vi "Bank of Parallel Filters.vi"() -> ()   [LabVIEW 2025]
uses:
  <vilib>/Analysis/1siggen.llb/Ramp Pattern by Samples.vi
  <vilib>/Analysis/2dsp.llb/Complex FFT.vi
  <vilib>/Analysis/baseanly.llb/Mean (CDB).vi
  <vilib>/Analysis/NI_AALPro.lvlib
  <vilib>/Analysis/NI_AALBase.lvlib
panel:
  in  "Cylcles Per Period":dbl=13.0 min=0.0 max=200.0 format="%#_13g"
  in  "Active Percent":dbl=100.0 min=0.0 max=100.0 step=1.0 format="%03.0f"
  in  "Offset":i32 min=0 max=100 step=1
  out "The Signal":dbl[](graph)
  out "The Spectrum":dbl[](graph)
  out "Parralell Filters":dbl[](graph)
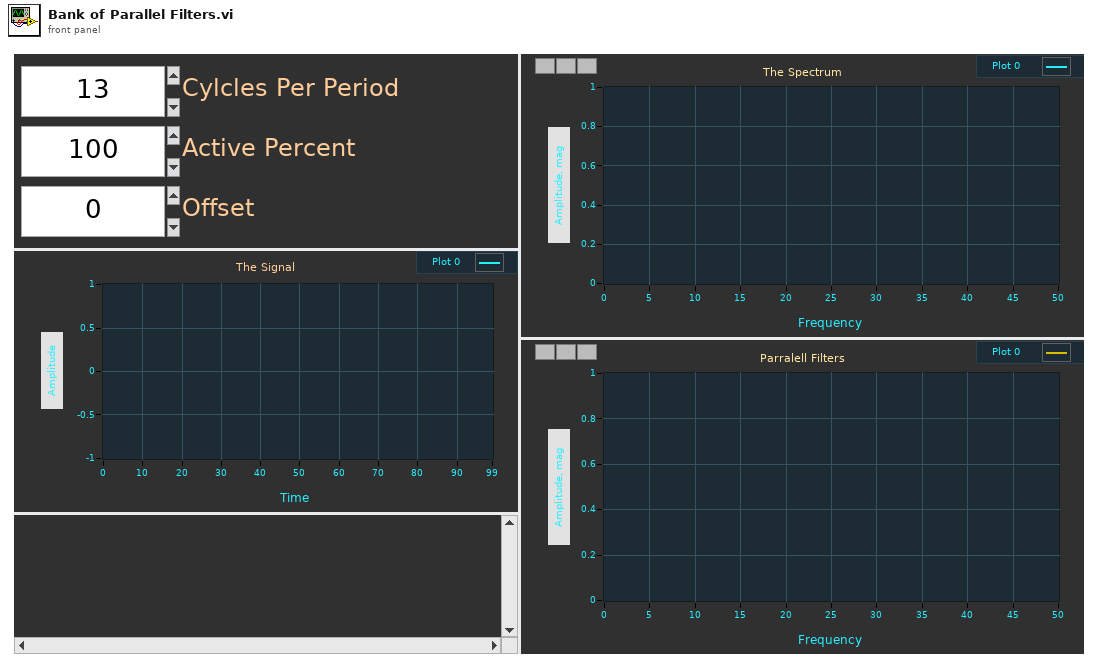
[diagram p1: front panel]
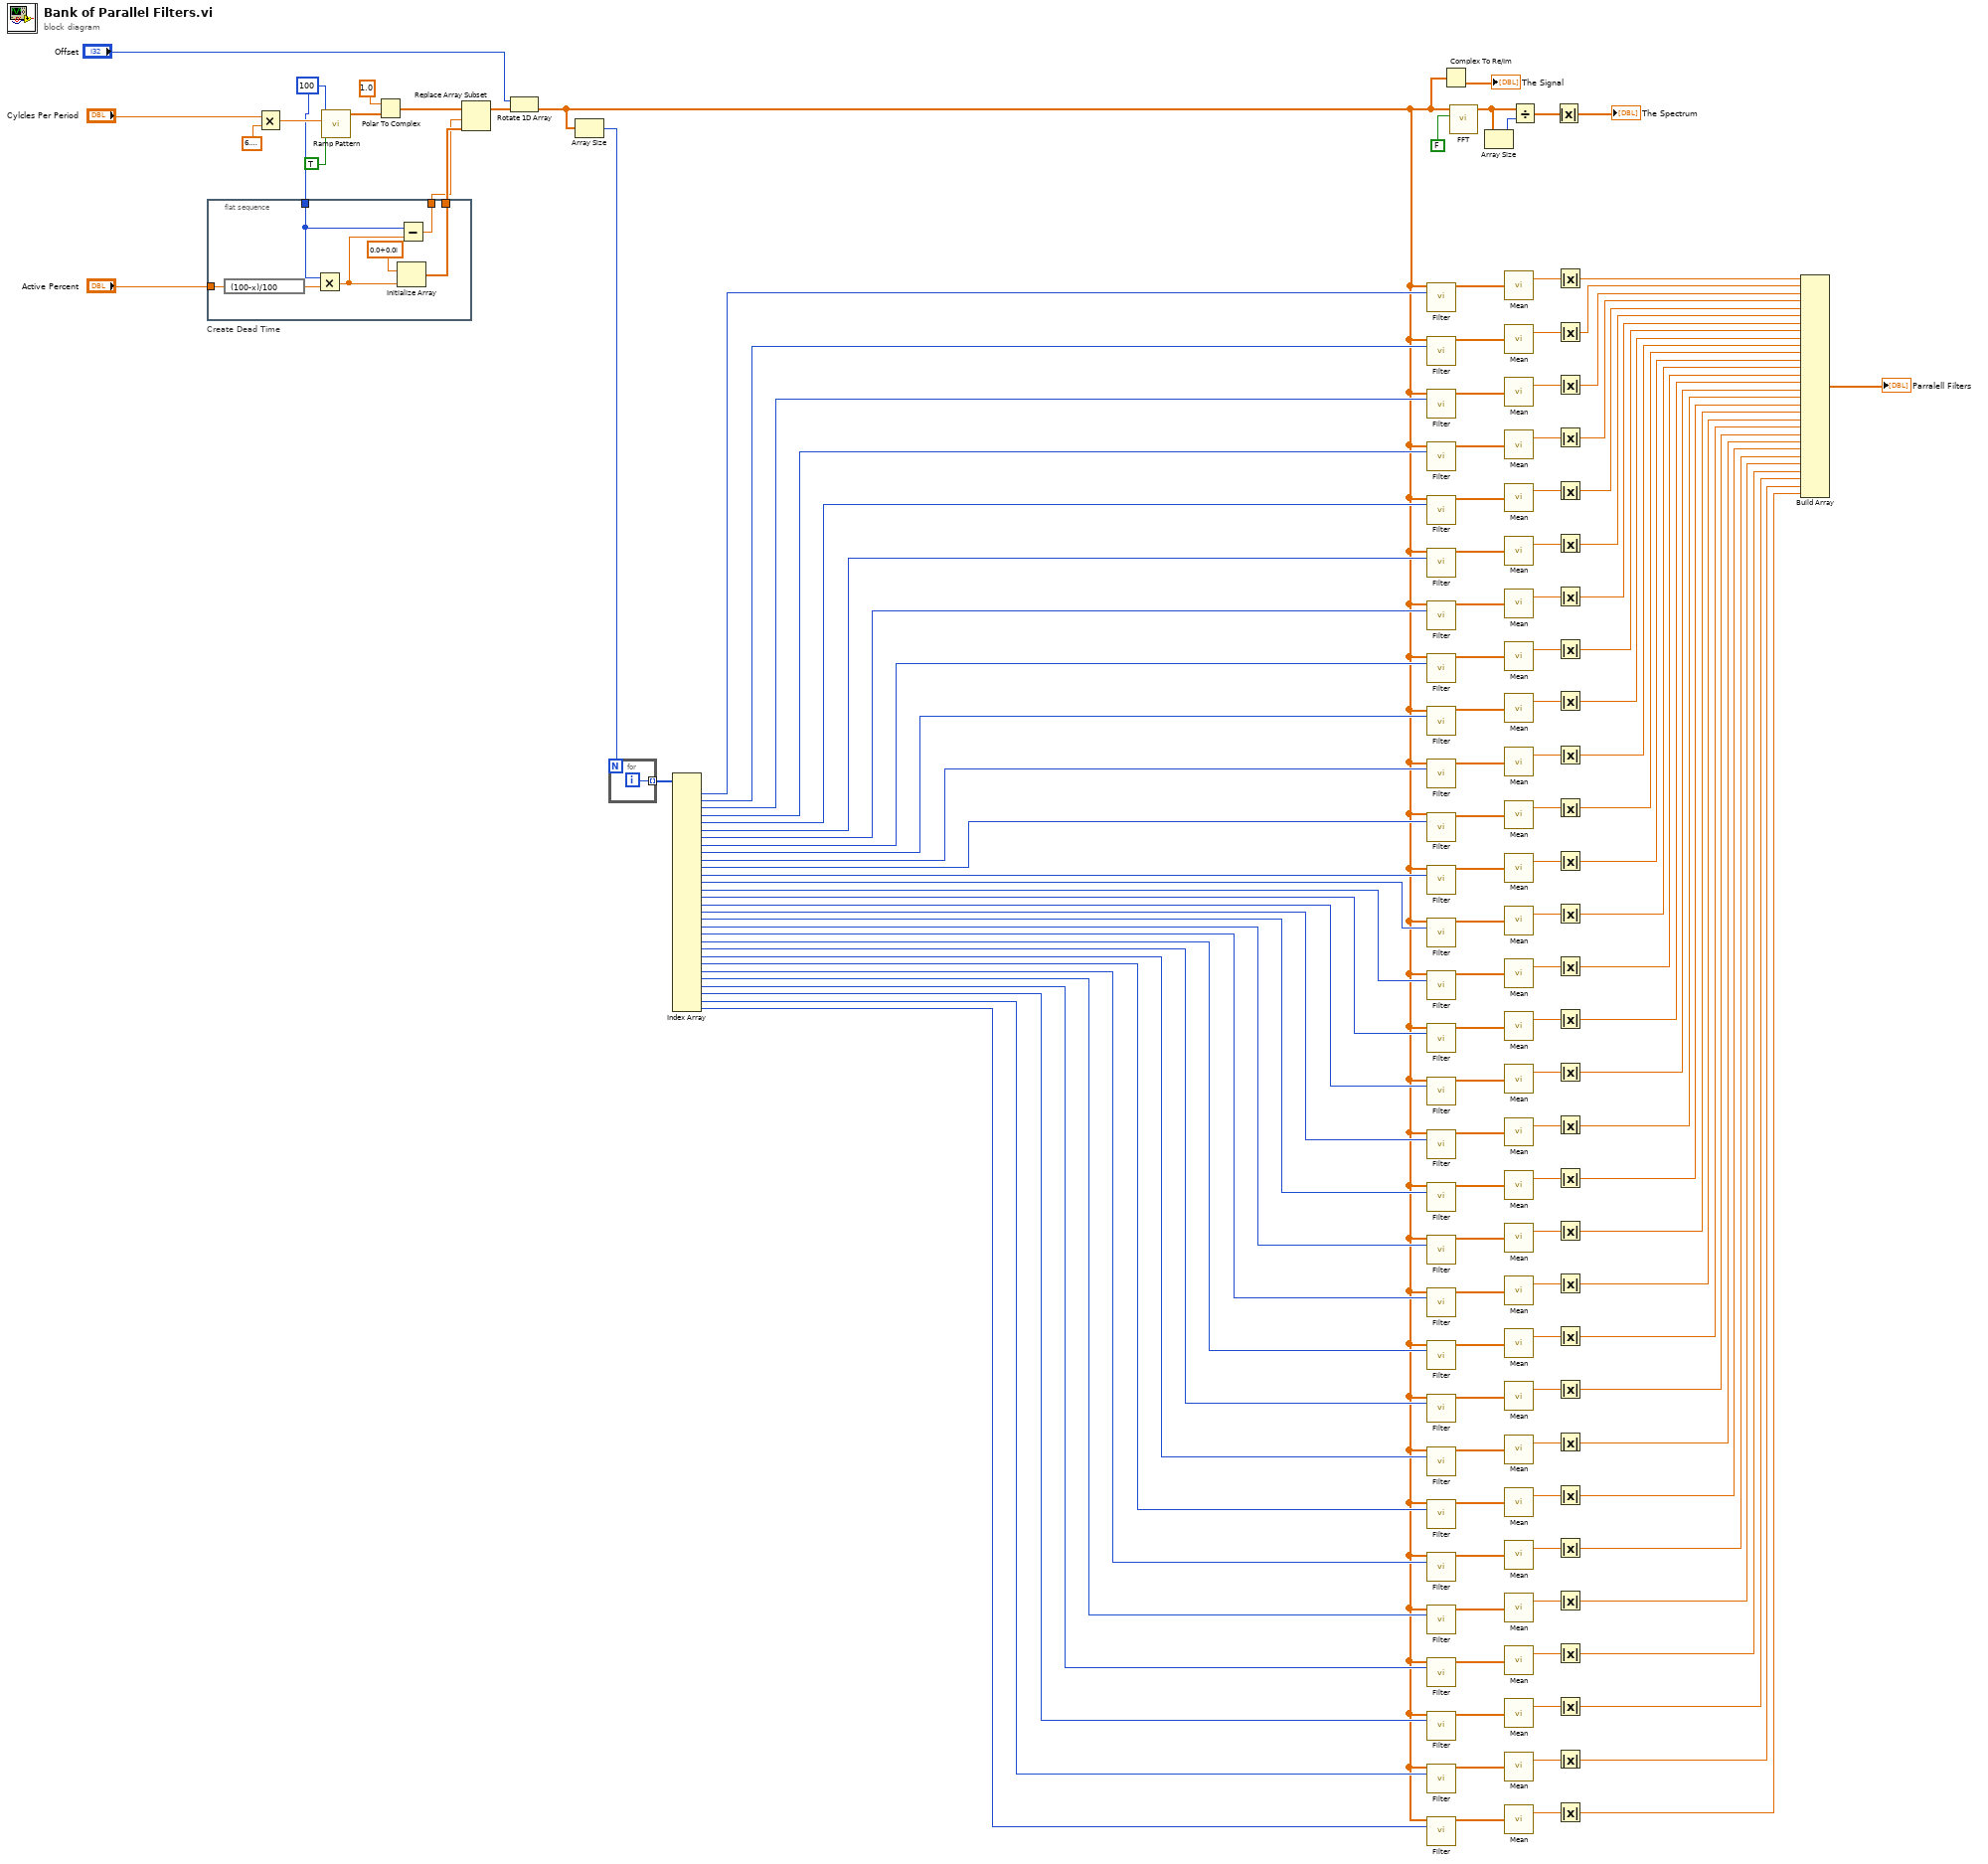
[diagram p0: block diagram]
diagram:
  w127 = 100 ("element")
  n1 = flat-sequence "Create Dead Time" {
    tunnel: "Active Percent" -> [w149]
    tunnel: [w147] -> w129
    tunnel: w127 -> [w146]
    tunnel: [w144] -> w126
    frame #0 {
      n2 = expression code="(100-x)/100"(w149) -> (w148:dbl)
      n3 = Multiply(x=w146, y=w148) -> (x*y=w145:dbl)
      n4 = Initialize Array(cdb 0.0+0.0i ("element"), w145) -> (w147:cdb[])
      n5 = Subtract(x=w146, y=w145) -> (x-y=w144:dbl)
    }
  }
  n6 = Multiply(x="Cylcles Per Period", y=6.283185307179586) -> (x*y=w143:dbl)
  n7 = call-poly <vilib>:"Ramp Pattern.vi"("exclude end?"=TRUE, "end"=w143, "samples"=w127) -> ("Ramp Pattern"=w139:dbl[])  [unwired: 7 in, 1 out]
  n8 = Polar To Complex(1:w139, 2:1.0 ("cycles")) -> (0:w130:cdb[])
  n9 = Replace Array Subset(array=w130, new element=w129, index=w126) -> (w128:cdb[])
  n10 = Rotate 1D Array(1:w128, 2:"Offset") -> (0:w1:cdb[])
  n11 = Array Size(array=w1) -> (size(s)=w124:i32)
  n12 = for {
    N: w124 -> [_]
    tunnel: [w151] -> w123 mode=indexing
    i -> [w151]
  }
  n13 = Index Array(array=w123) -> (element #1=w122:i32, element #2=w121:i32, element #3=w120:i32, element #4=w119:i32, element #5=w118:i32, element #6=w117:i32, element #7=w116:i32, element #8=w115:i32, element #9=w114:i32, element #10=w113:i32, element #11=w112:i32, element #12=w111:i32, element #13=w110:i32, element #14=w109:i32, element #15=w108:i32, element #16=w107:i32, element #17=w106:i32, element #18=w105:i32, element #19=w104:i32, element #20=w103:i32, element #21=w102:i32, element #22=w101:i32, element #23=w100:i32, element #24=w99:i32, element #25=w98:i32, element #26=w97:i32, element #27=w96:i32, element #28=w95:i32, element #29=w94:i32, element #30=w93:i32)  [unwired: 30 in]
  n14 = call "Filter.vi"("Array"=w1, "Numeric"=w122) -> ("mean"=w92:cdb[])  [unwired: 13 in]
  n15 = call "Filter.vi"("Array"=w1, "Numeric"=w121) -> ("mean"=w88:cdb[])  [unwired: 13 in]
  n16 = call "Filter.vi"("Array"=w1, "Numeric"=w120) -> ("mean"=w85:cdb[])  [unwired: 13 in]
  n17 = call "Filter.vi"("Array"=w1, "Numeric"=w119) -> ("mean"=w84:cdb[])  [unwired: 13 in]
  n18 = call "Filter.vi"("Array"=w1, "Numeric"=w118) -> ("mean"=w79:cdb[])  [unwired: 13 in]
  n19 = call "Filter.vi"("Array"=w1, "Numeric"=w117) -> ("mean"=w78:cdb[])  [unwired: 13 in]
  n20 = call "Filter.vi"("Array"=w1, "Numeric"=w116) -> ("mean"=w77:cdb[])  [unwired: 13 in]
  n21 = call "Filter.vi"("Array"=w1, "Numeric"=w115) -> ("mean"=w76:cdb[])  [unwired: 13 in]
  n22 = call "Filter.vi"("Array"=w1, "Numeric"=w114) -> ("mean"=w67:cdb[])  [unwired: 13 in]
  n23 = call "Filter.vi"("Array"=w1, "Numeric"=w113) -> ("mean"=w66:cdb[])  [unwired: 13 in]
  n24 = call "Filter.vi"("Array"=w1, "Numeric"=w112) -> ("mean"=w65:cdb[])  [unwired: 13 in]
  n25 = call "Filter.vi"("Array"=w1, "Numeric"=w111) -> ("mean"=w64:cdb[])  [unwired: 13 in]
  n26 = call "Filter.vi"("Array"=w1, "Numeric"=w110) -> ("mean"=w63:cdb[])  [unwired: 13 in]
  n27 = call "Filter.vi"("Array"=w1, "Numeric"=w109) -> ("mean"=w62:cdb[])  [unwired: 13 in]
  n28 = call "Filter.vi"("Array"=w1, "Numeric"=w108) -> ("mean"=w61:cdb[])  [unwired: 13 in]
  n29 = call "Filter.vi"("Array"=w1, "Numeric"=w107) -> ("mean"=w60:cdb[])  [unwired: 13 in]
  n30 = call "Filter.vi"("Array"=w1, "Numeric"=w106) -> ("mean"=w45:cdb[])  [unwired: 13 in]
  n31 = call "Filter.vi"("Array"=w1, "Numeric"=w105) -> ("mean"=w44:cdb[])  [unwired: 13 in]
  n32 = call "Filter.vi"("Array"=w1, "Numeric"=w104) -> ("mean"=w43:cdb[])  [unwired: 13 in]
  n33 = call "Filter.vi"("Array"=w1, "Numeric"=w103) -> ("mean"=w42:cdb[])  [unwired: 13 in]
  n34 = call "Filter.vi"("Array"=w1, "Numeric"=w102) -> ("mean"=w41:cdb[])  [unwired: 13 in]
  n35 = call "Filter.vi"("Array"=w1, "Numeric"=w101) -> ("mean"=w40:cdb[])  [unwired: 13 in]
  n36 = call "Filter.vi"("Array"=w1, "Numeric"=w100) -> ("mean"=w39:cdb[])  [unwired: 13 in]
  n37 = call "Filter.vi"("Array"=w1, "Numeric"=w99) -> ("mean"=w38:cdb[])  [unwired: 13 in]
  n38 = call "Filter.vi"("Array"=w1, "Numeric"=w98) -> ("mean"=w37:cdb[])  [unwired: 13 in]
  n39 = call "Filter.vi"("Array"=w1, "Numeric"=w97) -> ("mean"=w36:cdb[])  [unwired: 13 in]
  n40 = call "Filter.vi"("Array"=w1, "Numeric"=w96) -> ("mean"=w35:cdb[])  [unwired: 13 in]
  n41 = call "Filter.vi"("Array"=w1, "Numeric"=w95) -> ("mean"=w34:cdb[])  [unwired: 13 in]
  n42 = call "Filter.vi"("Array"=w1, "Numeric"=w94) -> ("mean"=w33:cdb[])  [unwired: 13 in]
  n43 = call "Filter.vi"("Array"=w1, "Numeric"=w93) -> ("mean"=w32:cdb[])  [unwired: 13 in]
  n44 = Complex To Re/Im(x + iy=w1) -> (y=→"The Signal":dbl[])  [unwired: 1 out]
  n45 = call-poly <vilib>:"FFT.vi"("shift?"=FALSE, "X"=w1) -> ("FFT {X}"=w134:cdb[])  [unwired: 8 in, 1 out]
  n46 = Array Size(array=w134) -> (size(s)=w133:i32)
  n47 = call-poly <vilib>:"Mean.vi"("X"=w92) -> ("mean"=w91:cdb)  [unwired: 1 out]
  n48 = call-poly <vilib>:"Mean.vi"("X"=w88) -> ("mean"=w89:cdb)  [unwired: 1 out]
  n49 = call-poly <vilib>:"Mean.vi"("X"=w85) -> ("mean"=w86:cdb)  [unwired: 1 out]
  n50 = call-poly <vilib>:"Mean.vi"("X"=w84) -> ("mean"=w87:cdb)  [unwired: 1 out]
  n51 = call-poly <vilib>:"Mean.vi"("X"=w79) -> ("mean"=w80:cdb)  [unwired: 1 out]
  n52 = call-poly <vilib>:"Mean.vi"("X"=w78) -> ("mean"=w81:cdb)  [unwired: 1 out]
  n53 = call-poly <vilib>:"Mean.vi"("X"=w77) -> ("mean"=w83:cdb)  [unwired: 1 out]
  n54 = call-poly <vilib>:"Mean.vi"("X"=w76) -> ("mean"=w82:cdb)  [unwired: 1 out]
  n55 = call-poly <vilib>:"Mean.vi"("X"=w67) -> ("mean"=w68:cdb)  [unwired: 1 out]
  n56 = call-poly <vilib>:"Mean.vi"("X"=w66) -> ("mean"=w69:cdb)  [unwired: 1 out]
  n57 = call-poly <vilib>:"Mean.vi"("X"=w65) -> ("mean"=w71:cdb)  [unwired: 1 out]
  n58 = call-poly <vilib>:"Mean.vi"("X"=w64) -> ("mean"=w70:cdb)  [unwired: 1 out]
  n59 = call-poly <vilib>:"Mean.vi"("X"=w63) -> ("mean"=w75:cdb)  [unwired: 1 out]
  n60 = call-poly <vilib>:"Mean.vi"("X"=w62) -> ("mean"=w74:cdb)  [unwired: 1 out]
  n61 = call-poly <vilib>:"Mean.vi"("X"=w61) -> ("mean"=w72:cdb)  [unwired: 1 out]
  n62 = call-poly <vilib>:"Mean.vi"("X"=w60) -> ("mean"=w73:cdb)  [unwired: 1 out]
  n63 = call-poly <vilib>:"Mean.vi"("X"=w45) -> ("mean"=w46:cdb)  [unwired: 1 out]
  n64 = call-poly <vilib>:"Mean.vi"("X"=w44) -> ("mean"=w47:cdb)  [unwired: 1 out]
  n65 = call-poly <vilib>:"Mean.vi"("X"=w43) -> ("mean"=w49:cdb)  [unwired: 1 out]
  n66 = call-poly <vilib>:"Mean.vi"("X"=w42) -> ("mean"=w48:cdb)  [unwired: 1 out]
  n67 = call-poly <vilib>:"Mean.vi"("X"=w41) -> ("mean"=w53:cdb)  [unwired: 1 out]
  n68 = call-poly <vilib>:"Mean.vi"("X"=w40) -> ("mean"=w52:cdb)  [unwired: 1 out]
  n69 = call-poly <vilib>:"Mean.vi"("X"=w39) -> ("mean"=w50:cdb)  [unwired: 1 out]
  n70 = call-poly <vilib>:"Mean.vi"("X"=w38) -> ("mean"=w51:cdb)  [unwired: 1 out]
  n71 = call-poly <vilib>:"Mean.vi"("X"=w37) -> ("mean"=w59:cdb)  [unwired: 1 out]
  n72 = call-poly <vilib>:"Mean.vi"("X"=w36) -> ("mean"=w58:cdb)  [unwired: 1 out]
  n73 = call-poly <vilib>:"Mean.vi"("X"=w35) -> ("mean"=w56:cdb)  [unwired: 1 out]
  n74 = call-poly <vilib>:"Mean.vi"("X"=w34) -> ("mean"=w57:cdb)  [unwired: 1 out]
  n75 = call-poly <vilib>:"Mean.vi"("X"=w33) -> ("mean"=w54:cdb)  [unwired: 1 out]
  n76 = call-poly <vilib>:"Mean.vi"("X"=w32) -> ("mean"=w55:cdb)  [unwired: 1 out]
  n77 = Divide(x=w134, y=w133) -> (x/y=w135:cdb[])
  n78 = Absolute Value(x=w135) -> (abs(x)=→"The Spectrum":dbl[])
  n79 = Absolute Value(x=w91) -> (abs(x)=w90:dbl)
  n80 = Absolute Value(x=w89) -> (abs(x)=w31:dbl)
  n81 = Absolute Value(x=w86) -> (abs(x)=w30:dbl)
  n82 = Absolute Value(x=w87) -> (abs(x)=w29:dbl)
  n83 = Absolute Value(x=w80) -> (abs(x)=w28:dbl)
  n84 = Absolute Value(x=w81) -> (abs(x)=w27:dbl)
  n85 = Absolute Value(x=w83) -> (abs(x)=w26:dbl)
  n86 = Absolute Value(x=w82) -> (abs(x)=w25:dbl)
  n87 = Absolute Value(x=w68) -> (abs(x)=w24:dbl)
  n88 = Absolute Value(x=w69) -> (abs(x)=w23:dbl)
  n89 = Absolute Value(x=w71) -> (abs(x)=w22:dbl)
  n90 = Absolute Value(x=w70) -> (abs(x)=w21:dbl)
  n91 = Absolute Value(x=w75) -> (abs(x)=w20:dbl)
  n92 = Absolute Value(x=w74) -> (abs(x)=w19:dbl)
  n93 = Absolute Value(x=w72) -> (abs(x)=w18:dbl)
  n94 = Absolute Value(x=w73) -> (abs(x)=w17:dbl)
  n95 = Absolute Value(x=w46) -> (abs(x)=w16:dbl)
  n96 = Absolute Value(x=w47) -> (abs(x)=w15:dbl)
  n97 = Absolute Value(x=w49) -> (abs(x)=w14:dbl)
  n98 = Absolute Value(x=w48) -> (abs(x)=w13:dbl)
  n99 = Absolute Value(x=w53) -> (abs(x)=w12:dbl)
  n100 = Absolute Value(x=w52) -> (abs(x)=w11:dbl)
  n101 = Absolute Value(x=w50) -> (abs(x)=w10:dbl)
  n102 = Absolute Value(x=w51) -> (abs(x)=w9:dbl)
  n103 = Absolute Value(x=w59) -> (abs(x)=w8:dbl)
  n104 = Absolute Value(x=w58) -> (abs(x)=w7:dbl)
  n105 = Absolute Value(x=w56) -> (abs(x)=w6:dbl)
  n106 = Absolute Value(x=w57) -> (abs(x)=w5:dbl)
  n107 = Absolute Value(x=w54) -> (abs(x)=w4:dbl)
  n108 = Absolute Value(x=w55) -> (abs(x)=w3:dbl)
  n109 = Build Array(w90, w31, w30, w29, w28, w27, w26, w25, w24, w23, w22, w21, w20, w19, w18, w17, w16, w15, w14, w13, w12, w11, w10, w9, w8, w7, w6, w5, w4, w3) -> (→"Parralell Filters":dbl[])
